vi "Does acquisition repeat.vi"(8 "error in (no error)":errorcluster, 11 "Measurement in":refnum<class "Measurement.lvclass">) -> (0 "error out":errorcluster, 3 "Measurement out":refnum<class "Measurement.lvclass">)   [LabVIEW 2015, in "Measurement Actor.lvlib" / "Measurement.lvclass"]
uses:
  Measurement.lvclass
  <vilib>/ActorFramework/Actor/Actor.lvclass/Actor.ctl
  <vilib>/ActorFramework/Message Enqueuer/Message Enqueuer.lvclass/Message Enqueuer.ctl
  <vilib>/ActorFramework/Message Enqueuer/Enqueue.vi
  <vilib>/ActorFramework/Message Enqueuer/Init from Existing Queue.vi
  <vilib>/ActorFramework/Message Priority Queue/Priority Enqueue.vi
  Messages/Measure Msg/Measure Msg.lvclass
  Messages/Acquire Continuously Msg/Acquire Continuously Msg.lvclass
  <vilib>/ActorFramework/Message Enqueuer/Message Enqueuer.lvclass
  <vilib>/ActorFramework/Actor/Actor.lvclass
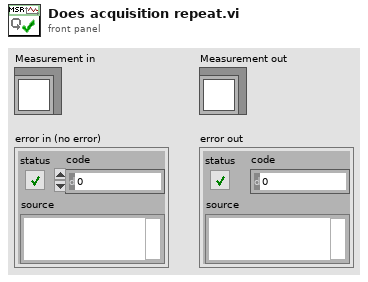
[diagram p1: front panel]
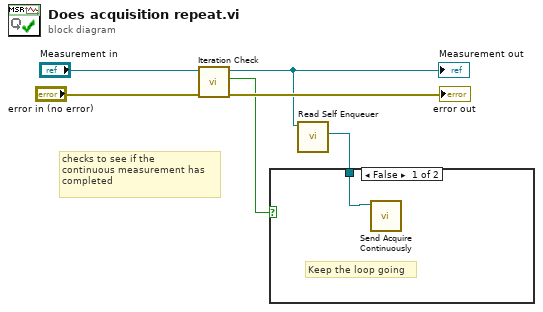
[diagram p0: block diagram]
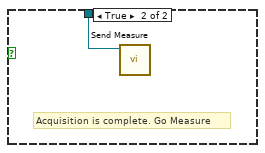
[diagram p2: hidden frame]
diagram:
  # "checks to see if the \ncontinuous measurement has\ncompleted"
  n1 = call "Iteration Check.vi"("error in (no error)"="error in (no error)", "Measurement in"="Measurement in") -> ("error out"=→"error out":errorcluster, "Done?"=w2:bool, "Measurement out"=w1:refnum<class "Measurement.lvclass">)  [unwired: 7 in]
  "Measurement out" <- w1
  n2 = call <vilib>:"Read Self Enqueuer.vi"("Actor"=w1) -> ("Self Enqueuer"=w3:refnum<class "Message Enqueuer.lvclass">)  [unwired: 10 in]
  n3 = case shown="False" w2 {
    tunnel: w3 -> [w7 w8]
    frame False {
      # "Keep the loop going"
      n4 = call "Send Acquire Continuously.vi"("Message Enqueuer"=w7) -> ()  [unwired: 9 in, 2 out]
    }
    frame True {
      # "Acquisition is complete. Go Measure"
      n5 = call "Send Measure.vi"("Message Enqueuer in"=w8) -> ()  [unwired: 9 in, 2 out]
    }
  }
